vi "Platypi Complementary Filter.vi"() -> ()   [LabVIEW 2014]
doc: "I. Description:\nThis example demonstrates how to output a single Voltage Update (Sample) to an Analog Output Channel.\n\nII. Instructions for Running:\n1. Select the Physical Channel to correspond to where your signal is output on the DAQ device.\n2. Enter the Minimum and Maximum Voltage Ranges\nNote: Use the Acq One Sample example to verify you are generating the correct output on the DAQ device\n\nIII. Block Diagram Steps:\n1. Create an Analog Output Voltage Channel\n2. Use the Write VI to Output 1 Sample to 1 Channel on the Data\nAcquisition Card. \n3. Call the Clear Task VI to clear the Task.\n4. Use the popup dialog box to display an error if any. \n\nIV. I/O Connections Overview:\nMake sure your signal output terminal matches the Physical Channel I/O Control. For further connection information, refer to your hardware reference manual."
uses:
  <vilib>/picture/3D Picture Control/NI_3D Picture Control.lvlib
  <vilib>/Rock Robotics/SystemInterfaces/spilib/spi_bus.ctl
  Sensors/ADXRS450/ADXRS453_Global.vi
panel:
  out "Data Display":T1(graph)
  in  "Filter Coefficient a":dbl(slide)=0.7473684210526316 scale=0.0..1.0
  in  "Stop":bool
  in  "Initialize Accel":bool
  in  "Initialize Gyro":bool
  in  "Sensitivity (mV/g)":dbl=330.0
  out "Time Constant (s)":dbl
  out "Gyro":refnum<vi>(3d-picture)
  out "Accelerometer":refnum<vi>(3d-picture)
  out "Filtered Accelerometer & Gyro":refnum<vi>(3d-picture)
  # "myComplementary Filter"
  # "Chart Information"
  # "Channel Parameters"
  # "Gyro Parameters"
  # "Accelerometer Parameters"
  # "Complementary Filter Parameters"
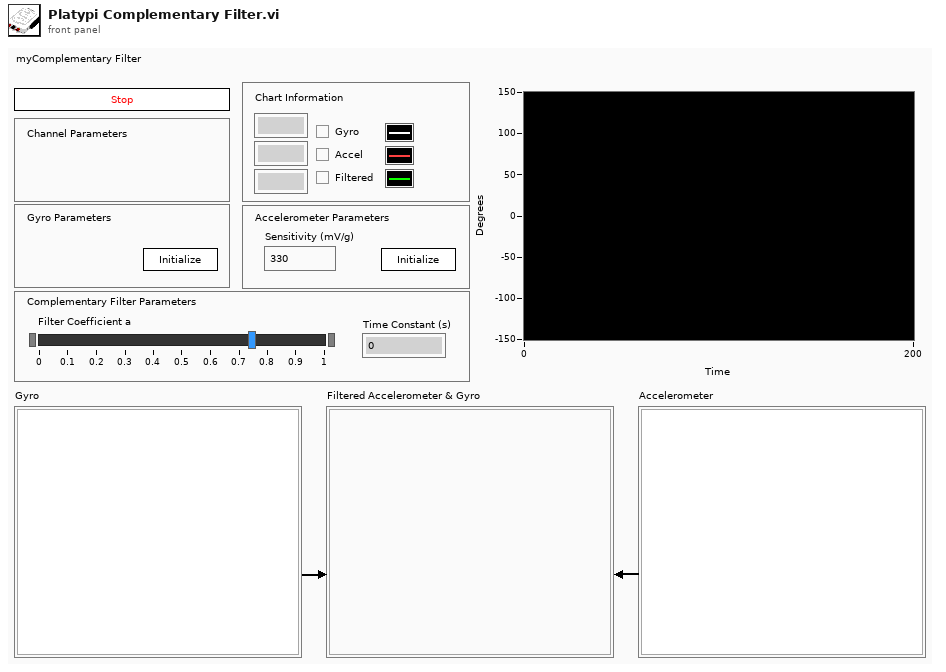
[diagram p1: front panel]
types:
  T1 = cluster{"Rate of turn (°/s)":dbl, "Angle from horizontal (°)":dbl, "Filtered":dbl}
  T2 = typedef "spi_bus.ctl" = enum16{"SPI On-Board, CS0", "SPI On-Board, CS1", "SPI On-Board, CS2", "SPI On-Board, CS3", "SPI MXP", "Invalid"}
  T3 = cluster{"Red":sgl, "Green":sgl, "Blue":sgl, "Alpha":sgl}
  T4 = typedef "WPI_SPIDevRef.ctl" = cluster{"DevStatus":errorcluster, "Handle":i32, "Controller":T5, "SPI Bus":T2}
  T5 = typedef "FPGA_TypedefDigitalModule.ctl" = enum16{"Controller 1"}
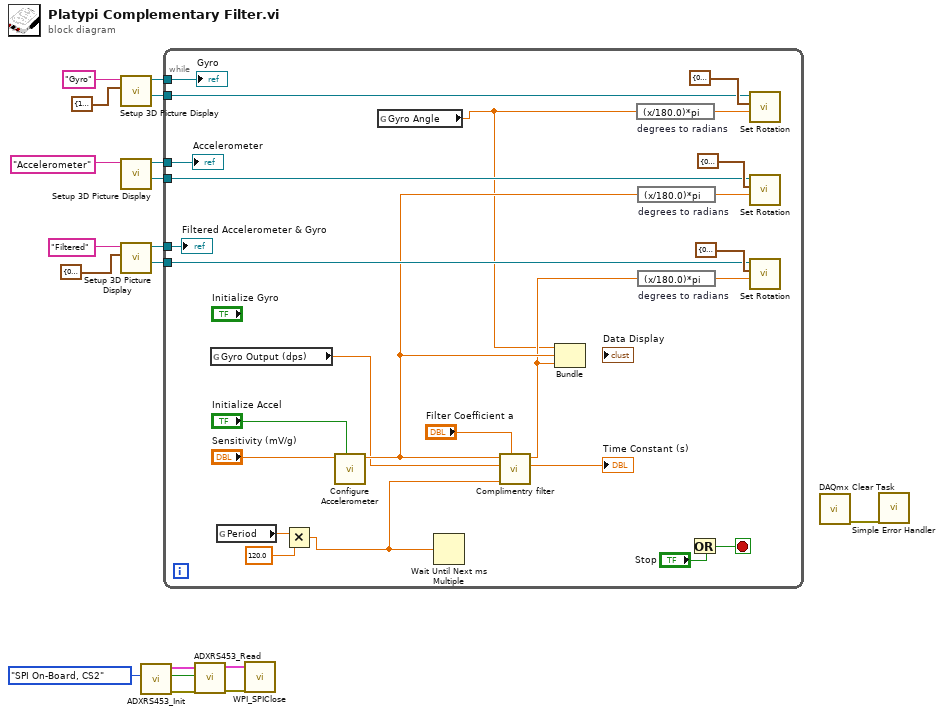
[diagram p0: block diagram]
diagram:
  n1 = call "Setup 3D Picture Display.vi"("Color"=T3 {"Red"=1.0, "Green"=1.0, "Blue"=1.0, "Alpha"=1.0}, "Name"="Gyro") -> ("SceneObject out"=w17:refnum<vi>, "Scene:New Object"=w16:refnum<vi>)  [unwired: 8 in]
  n2 = call "Setup 3D Picture Display.vi"("Name"="Accelerometer") -> ("SceneObject out"=w13:refnum<vi>, "Scene:New Object"=w14:refnum<vi>)  [unwired: 9 in]
  n3 = call "Setup 3D Picture Display.vi"("Color"=T3 {"Red"=0.0, "Green"=1.0, "Blue"=0.0, "Alpha"=1.0}, "Name"="Filtered") -> ("SceneObject out"=w10:refnum<vi>, "Scene:New Object"=w11:refnum<vi>)  [unwired: 8 in]
  n4 = call "ADXRS453_Init.vi"("SPI Bus"=spi_bus."SPI On-Board, CS2") -> ("Error Out"=w4:errorcluster, "Gyro Detected?"=w5:bool, "ADXRS453 Ref Out"=w6:T4)  [unwired: 8 in]
  n5 = while {
    tunnel: w11 -> [w42]
    tunnel: w10 -> [w39]
    tunnel: w14 -> [w38]
    tunnel: w13 -> [w35]
    tunnel: w17 -> [w30]
    tunnel: w16 -> [w29]
    stop <- w43 stop-if-true
    n6 = global read "ADXRS453_Global.vi" "Gyro Output (dps)"() -> (w19:dbl)
    n7 = global read "ADXRS453_Global.vi" "Period"() -> (w23:dbl)
    n8 = Multiply(x=w23, y=120.0) -> (x*y=w21:dbl)
    n9 = call "Configure Accelerometer.vi"("Initialize"="Initialize Accel", "Sensitivity (mV/g)"="Sensitivity (mV/g)") -> ("Angle from horizontal (°)"=w25:dbl)  [unwired: 9 in]
    n10 = global read "ADXRS453_Global.vi" "Gyro Angle"() -> (w20:dbl)
    n11 = Wait Until Next ms Multiple(millisecond multiple=w21) -> ()  [unwired: 1 out]
    n12 = call "Complimentry filter.vi"("Filter Coefficient a"="Filter Coefficient a", "dt (ms)"=w21, "Gyro (degrees/second)"=w19, "Accelerometer (degrees)"=w25) -> ("timeConstant"=→"Time Constant (s)":dbl, "Filtered"=w24:dbl)  [unwired: 6 in]
    n13 = Bundle("Gyro Angle"=w20, "Angle from horizontal (°)"=w25, "Filtered"=w24) -> ()  [unwired: 1 in, 1 out]
    n14 = expression code="(x/180.0)*pi" "degrees to radians"(w20) -> (w33:dbl)
    n15 = expression code="(x/180.0)*pi" "degrees to radians"(w25) -> (w37:dbl)
    n16 = expression code="(x/180.0)*pi" "degrees to radians"(w24) -> (w40:dbl)
    n17 = Or(y="Stop") -> (x .or. y?=w43:bool)  [unwired: 1 in]
    n18 = call <vilib>:"Set Rotation.vi"("Angle"=w33, "Axis"=cluster{"X":sgl, "Y":sgl, "Z":sgl} {"X"=0.0, "Y"=1.0, "Z"=0.0}, "Scene Object"=w30) -> ()  [unwired: 7 in, 2 out]
    n19 = call <vilib>:"Set Rotation.vi"("Angle"=w37, "Axis"=cluster{"X":sgl, "Y":sgl, "Z":sgl} {"X"=0.0, "Y"=1.0, "Z"=0.0}, "Scene Object"=w35) -> ()  [unwired: 7 in, 2 out]
    n20 = call <vilib>:"Set Rotation.vi"("Angle"=w40, "Axis"=cluster{"X":sgl, "Y":sgl, "Z":sgl} {"X"=0.0, "Y"=1.0, "Z"=0.0}, "Scene Object"=w39) -> ()  [unwired: 7 in, 2 out]
    "Filtered Accelerometer & Gyro" <- w42
    "Accelerometer" <- w38
    "Gyro" <- w29
  }
  n21 = call "ADXRS453_Read.vi"("Error In"=w4, "Gyro Detected?"=w5, "ADXRS453 Ref In"=w6) -> ("Error Out"=w2:errorcluster, "ADXRS453 Ref Out"=w1:T4)  [unwired: 7 in]
  n22 = call <vilib>:"WPI_SPIClose.vi"("error in (no error)"=w2, "SPIDevRef"=w1) -> ()  [unwired: 9 in, 1 out]
  n23 = call <vilib>:"DAQmx Clear Task.vi"() -> ("error out"=w18:errorcluster)  [unwired: 15 in]
  n24 = call <vilib>:"Simple Error Handler.vi"("error in (no error)"=w18) -> ()  [unwired: 4 in, 5 out]
